vi "VI Name.vi"(10 "class name (\"\")":string, 11 "vi name":string) -> (3 "full VI name":string)   [LabVIEW 2017, in "DSF Core.lvlib"]
uses:
  DSF Core.lvlib
  Constants/Engine Library Name.vi
  Classes/Framework/Framework.lvclass
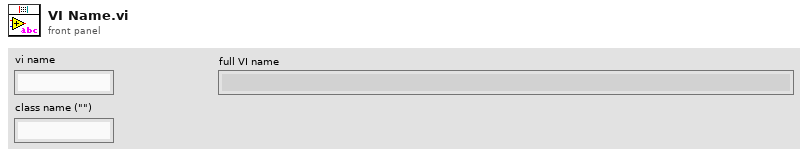
[diagram p1: front panel]
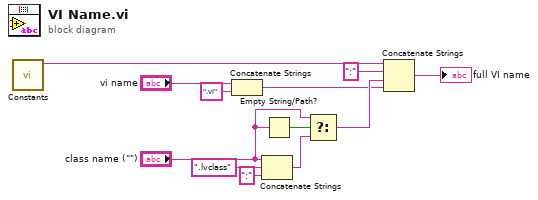
[diagram p0: block diagram]
diagram:
  n1 = call-poly "Constants.vi"() -> ("Engine Library Name"=w5:string)  [unwired: 11 in]
  n2 = Concatenate Strings("vi name", ".vi" ("string")) -> (w1:string)
  n3 = Concatenate Strings("class name (\"\")", ".lvclass" ("string"), ":" ("string")) -> (w10:string)
  n4 = Empty String/Path?(string/path="class name (\"\")") -> (empty?=w11:bool)
  n5 = Select(t="class name (\"\")", s=w11, f=w10) -> (s? t:f=w9:string)
  n6 = Concatenate Strings(w5, ":" ("string"), w9, w1) -> (→"full VI name":string)
